vi "UDP_SendData.vi"(5 "Remote Port":u16=33332, 7 "Remote MAC Address":string="00:00:00:00:00:00", 8 "error in":errorcluster, 10 "Parameters":string, 11 "Command":string) -> (0 "error out":errorcluster)   [LabVIEW 2014, in "hse-network.lvlib"]
doc: "____\nHAMPEL SOFTWARE ENGINEERING v0.7.0 (2018-07-16 18:12)"
uses:
  hse-network.lvlib
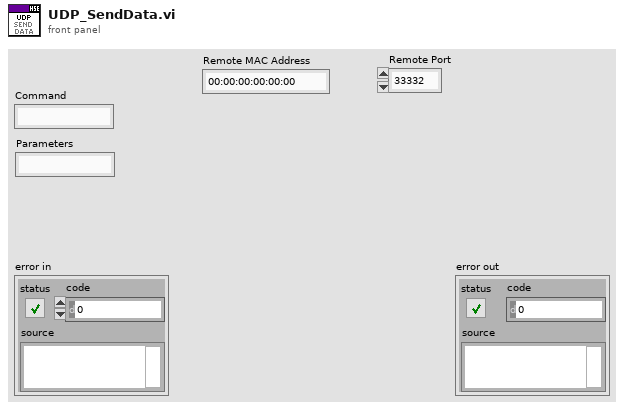
[diagram p1: front panel]
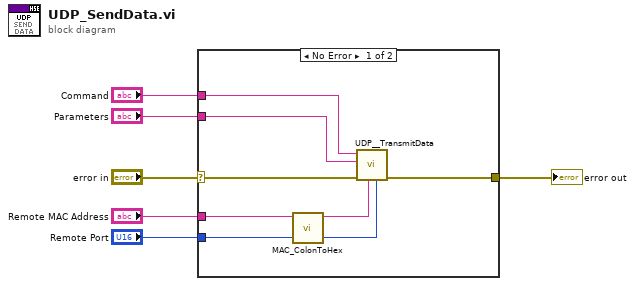
[diagram p0: block diagram]
diagram:
  n1 = case shown="No Error" "error in" {
    selector: "error in" -> [w12 w14]
    tunnel: "Remote Port" -> [w7 _]
    tunnel: "Command" -> [w13 _]
    tunnel: [w11 w14] -> w4
    tunnel: "Parameters" -> [w10 _]
    tunnel: "Remote MAC Address" -> [w9 _]
    frame No Error {
      n2 = call "MAC_ColonToHex.vi"("MAC Address (colon notation)"=w9) -> ("MAC Address (hex string)"=w8:string)  [unwired: 10 in]
      n3 = call "UDP__TransmitData.vi"("Remote Port"=w7, "Remote MAC Address (hex)"=w8, "error in"=w12, "Parameters"=w10, "Command"=w13) -> ("error out"=w11:errorcluster)  [unwired: 6 in]
    }
    frame Error {
    }
  }
  "error out" <- w4
